vi "RSZVB Set Reference.vi"(8 "error in (no error)":errorcluster {"code" format="%.0x"}, 10 "Reference (0: Internal)":i32(ring) items=["Internal", "External"], 11 "VISA session":refnum<visa-resource-name>) -> (0 "error out":errorcluster {"code" format="%.0x"}, 3 "dup VISA session":refnum<visa-resource-name>)   [LabVIEW 2011]
doc: "This VI selects the source of the reference oscillator signal.\n\nRemote-control command(s):\n[SENSe<Ch>:]ROSCillator[:SOURce] INTernal | EXTernal"
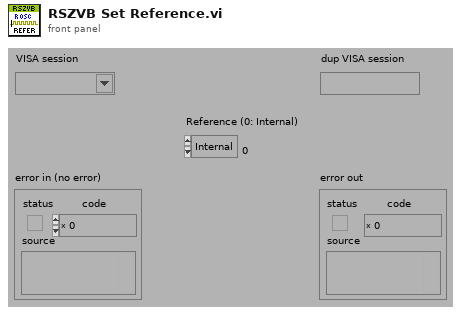
[diagram p1: front panel]
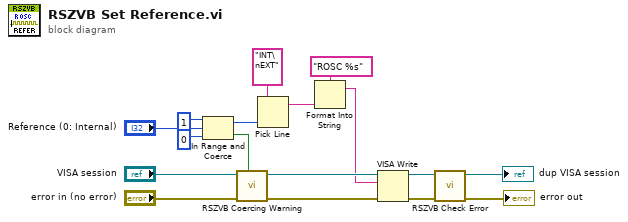
[diagram p0: block diagram]
diagram:
  n1 = In Range and Coerce(upper limit=1, x="Reference (0: Internal)", lower limit=0) -> (coerced(x)=w7:i32, In Range?=w10:bool)
  n2 = call "RSZVB Coercing Warning.vi"("In Range?"=w10, "error in (no error)"="error in (no error)", "VISA session"="VISA session") -> ("error out"=w13:errorcluster, "dup VISA session"=w14:refnum<visa-resource-name>)  [unwired: 7 in]
  n3 = Pick Line(multi-line string="INT\nEXT", line index=w7) -> (output string=w6:string)  [unwired: 1 in]
  n4 = Format Into String(format string="ROSC %s", w6) -> (resulting string=w9:string)  [unwired: 2 in, 1 out]
  n5 = VISA Write(VISA resource name=w14, write buffer=w9, error in (no error)=w13) -> (VISA resource name out=w11:refnum<visa-resource-name>, error out=w12:errorcluster)  [unwired: 1 out]
  n6 = call "RSZVB Check Error.vi"("error in (no error)"=w12, "VISA session"=w11) -> ("error out"=→"error out":errorcluster, "dup VISA session"=→"dup VISA session":refnum<visa-resource-name>)  [unwired: 8 in]
